vi "QA.vi"(8 "ERRIN":errorcluster caption="entrée d'erreur (pas d'erreur)", 10 "VISA":refnum<visa-resource-name>) -> (0 "ERROUT":errorcluster caption="sortie d'erreur", 2 "DATAOUT":string)   [LabVIEW 2020]
panel:
  # "<\\B20\\BE:(A\\CC\\A9:P\\D2\\C5SS\\C9\\CFN\\A0HAU\\D4\\C5\\8D\\n"
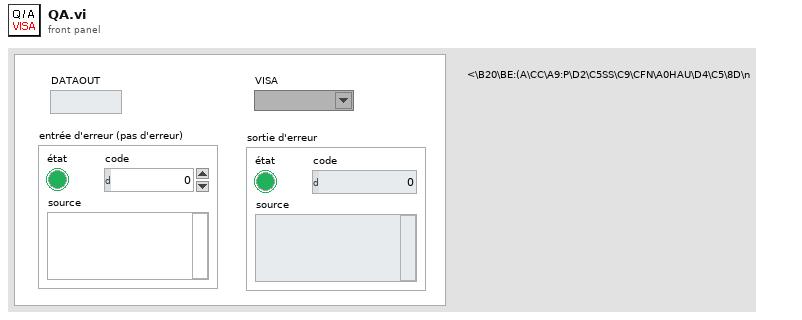
[diagram p1: front panel]
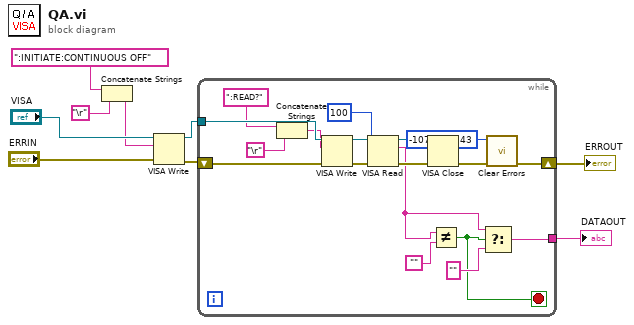
[diagram p0: block diagram]
diagram:
  n1 = Concatenate Strings(":INITIATE:CONTINUOUS OFF", "\r") -> (w3:string)
  n2 = VISA Write(VISA resource name="VISA", write buffer=w3, error in (no error)="ERRIN") -> (VISA resource name out=w2:refnum<visa-resource-name>, error out=w1:errorcluster)  [unwired: 1 out]
  n3 = while {
    tunnel: [w26] -> w8
    tunnel: w2 -> [w15]
    shift-right: [w11] -> w9
    shift-left: w1 -> [w16]
    stop <- w17 stop-if-true
    n4 = Concatenate Strings(":READ?", "\r") -> (w12:string)
    n5 = VISA Write(VISA resource name=w15, write buffer=w12, error in (no error)=w16) -> (VISA resource name out=w21:refnum<visa-resource-name>, error out=w23:errorcluster)  [unwired: 1 out]
    n6 = VISA Read(VISA resource name=w21, byte count=u32 100 ("nombre d'octets"), error in (no error)=w23) -> (VISA resource name out=w24:refnum<visa-resource-name>, read buffer=w18:string, error out=w25:errorcluster)  [unwired: 1 out]
    n7 = VISA Close(VISA resource name=w24, error in (no error)=w25) -> (error out=w27:errorcluster)
    n8 = Not Equal?(x=w18, y="") -> (x != y?=w17:bool)
    n9 = Select(t=w18, s=w17, f="") -> (s? t:f=w26:string)
    n10 = call <vilib>:"Clear Errors.vi"("error in (no error)"=w27, "specific error code to clear (0: all)"=-1073807343) -> ("error out"=w11:errorcluster)  [unwired: 4 in, 1 out]
  }
  "ERROUT" <- w9
  "DATAOUT" <- w8
